vi "getActionPanelPath.vi"(8 "error in (no error)":errorcluster, 11 "RampAction in":refnum<class "RampAction.lvclass">) -> (0 "error out":errorcluster, 2 "frontPanelPath":path, 3 "RampAction out":refnum<class "RampAction.lvclass">)   [LabVIEW 2011, in "Views.lvlib" / "ScriptEditor.lvlib" / "RampAction.lvclass"]
uses:
  RampAction.lvclass
  Tools/Filing/FileSystem/FileSystem.lvclass
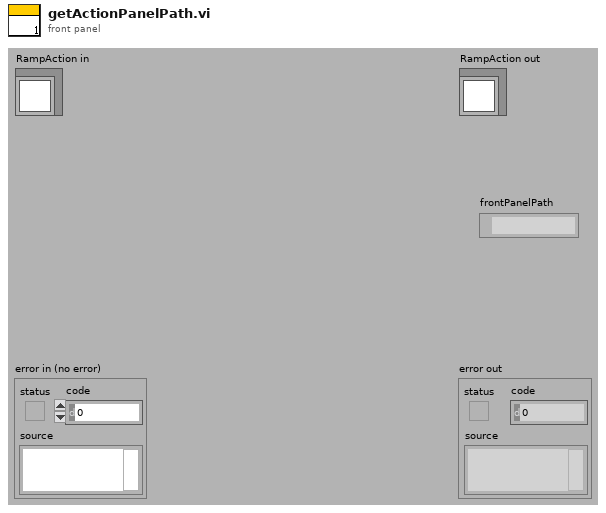
[diagram p1: front panel]
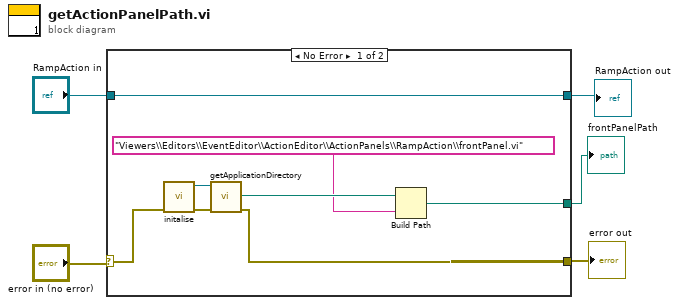
[diagram p0: block diagram]
diagram:
  n1 = case shown="No Error" "error in (no error)" {
    selector: "error in (no error)" -> [w11 w15]
    tunnel: [w7 w15] -> w4
    tunnel: "RampAction in" -> [w13 w14]
    tunnel: [w13 w14] -> w2
    tunnel: [w6 _] -> w1
    frame No Error {
      n2 = call "initalise.vi"("error in (no error)"=w11) -> ("error out"=w12:errorcluster, "FileSystem out"=w10:refnum<class "FileSystem.lvclass">)  [unwired: 9 in]
      n3 = call-dynamic "getApplicationDirectory.vi"("error in (no error)"=w12, "FileSystem.lvclass in"=w10) -> ("error out"=w7:errorcluster, "ApplicationDirectory"=w9:path)  [unwired: 7 in, 1 out]
      n4 = Build Path(base path=w9, name or relative path="Viewers\\Editors\\EventEditor\\ActionEditor\\ActionPanels\\RampAction\\frontPanel.vi") -> (appended path=w6:path)
    }
    frame Error {
    }
  }
  "error out" <- w4
  "RampAction out" <- w2
  "frontPanelPath" <- w1
